vi "oa_Process Order Power Spectrum (N Channels).vi"(0 "even angle signals":cluster{"r0":dbl, "dr":dbl, "Y":dbl[]}[](array[cluster]) {"r0" format="%.2p"; "dr" format="%.2p"; "Y" format="%.2f"}, 5 "channel info":T9[](array[typedef]) {"channel info"."pregain" format="%.2f"; "channel info"."weighting filter" items=["Linear", "A-weighting", "B-weighting", "C-weighting", "ITU-R 468-4", "Dolby", "CCITT", "C-message", "Wb", "Wc", "Wd", "We", "Wf", "Wh", "Wj", "Wk", "Wm", "AES17 20 kHz lowpass", "AES17 40 kHz lowpass", "AES17 20 kHz highpass", "AES17 40 kHz highpass"]; "channel info"."dB reference" format="%^.1e"; "channel info"."engineering units" items=["custom..."=0, "V"=1, "A"=21, "C"=30, "pC"=31, "s"=32, "-"=29, "Pa"=2, "N"=20, "g"=3, "m/s^2"=4, "m/s"=5, "m"=6, "mm/s"=12, "mm"=13, "micron/s"=14, "micron"=15, "in/s^2"=7, "in/s"=8, "in"=9, "mil/s"=10, "mil"=11, "rad/s^2"=16, "rad/s"=17, "rad"=18, "deg/s^2"=26, "deg/s"=27, "deg"=28, "RPM"=22, "cycle/s^2"=23, "Hz"=24, "cycle"=25, "strain"=19]; "channel info"."sensor sensitivity" format="%#_5f"}, 7 "spectrum settings":cluster{"window type":u32, "block size":i32}={"window type"=1, "block size"=400} {"block size" min=2; "window type" items=["None"=0, "Hanning"=1, "Hamming"=2, "Blackman-Harris"=3, "Exact Blackman"=4, "Blackman"=5, "Flat Top"=6, "4 Term B-Harris"=7, "7 Term B-Harris"=8, "Low Sidelobe"=9, "Gaussian"=62]}, 9 "averaging parameters":T11={"averaging mode"=enum."No averaging", "weighting mode"=enum."Exponential", "number of averages"=10, "linear mode"=enum."One shot"} {"number of averages" min=1 step=1}, 11 "error in":errorcluster, 12 "processing control in":T8(ring)) -> (2 "new spectrum available?":bool, 3 "averages completed":dbl, 4 "order power spectrum":T7(array[cluster]) {"order 0" format="%.2p"; "delta order" format="%.2p"; "magnitude" format="%.2f"}, 8 "averaging done":bool, 10 "spectrum info":T1[](array[typedef]) {"x-axis units" items=["Time (s)"=0, "Frequency-CB (Hz)"=1, "Frequency-CPB (Hz)"=1248, "Frequency-Arbitrary (Hz)"=2357, "Quefrency (s)"=2, "Revolutions (rev)"=3, "Order"=4, "Speed (RPM)"=11, "Speed (rad/s)"=21, "Index"=65535]; "weighting filter" items=["Linear", "A-weighting", "B-weighting", "C-weighting", "ITU-R 468-4", "Dolby", "CCITT", "C-message", "Wb", "Wc", "Wd", "We", "Wf", "Wh", "Wj", "Wk", "Wm", "AES17 20 kHz lowpass", "AES17 40 kHz lowpass", "AES17 20 kHz highpass", "AES17 40 kHz highpass"]; "dB reference [EU]" format="%.2f"; "engineering units" items=["custom..."=0, "V"=1, "A"=21, "C"=30, "pC"=31, "s"=32, "-"=29, "Pa"=2, "N"=20, "g"=3, "m/s^2"=4, "m/s"=5, "m"=6, "mm/s"=12, "mm"=13, "micron/s"=14, "micron"=15, "in/s^2"=7, "in/s"=8, "in"=9, "mil/s"=10, "mil"=11, "rad/s^2"=16, "rad/s"=17, "rad"=18, "deg/s^2"=26, "deg/s"=27, "deg"=28, "RPM"=22, "cycle/s^2"=23, "Hz"=24, "cycle"=25, "strain"=19]; "spectral info"."window" items=["None "=0, "Hanning"=1, "Hamming"=2, "Blackman-Harris"=3, "Exact Blackman"=4, "Blackman"=5, "Flat Top"=6, "4 Term B-Harris "=7, "7 Term B-Harris"=8, "Low Sidelobe"=9, "Force - Exponential"=10, "Gaussian"=62]}, 14 "processing control out":T8(ring), 15 "error out":errorcluster)   [LabVIEW 2017, in "SoundVib_Resampling.lvlib"]
uses:
  <vilib>/addons/Sound and Vibration/Order Analysis/Resample Order Tracking/SoundVib_Resampling.lvlib
  <vilib>/addons/_NISVFA/_Shared subVIs/Controls/svc_Resampled Channel Info.ctl
  <vilib>/addons/_NISVFA/_Shared subVIs/Controls/svc_Channel Info.ctl
  <vilib>/addons/_NISVFA/_Shared subVIs/Controls/svc_Engineering Units Text Ring.ctl
  <vilib>/addons/_NISVFA/_Shared subVIs/Controls/svc_Weighting Filter Text Ring.ctl
  <vilib>/addons/_NISVFA/_Shared subVIs/Controls/svc_Spectrum Info.ctl
  <vilib>/addons/_NISVFA/_Shared subVIs/Controls/svc_X-Axis Units.ctl
  <vilib>/addons/_NISVFA/_Shared subVIs/Controls/svc_Spectrum Type.ctl
  <vilib>/addons/_NISVFA/_Shared subVIs/Controls/svc_Complimentary Spectrum Units.ctl
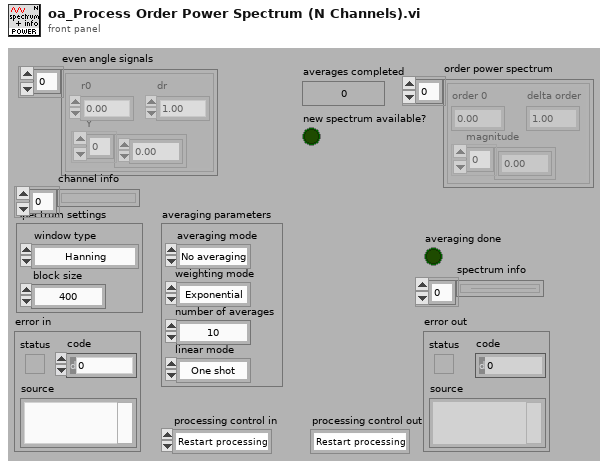
[diagram p1: front panel]
types:
  T1 = typedef "svc_Spectrum Info.ctl" = cluster{"channel name":string, "description":string, "x-axis units":T2, "spectral info":cluster{"spectrum type":T3, "linear/dB":enum16{"linear", "dB"}, "window":u16, "window size":i32, "FFT size":i32}, "engineering units":T4, "custom label":string, "dB reference [EU]":dbl, "peak units":enum16{"rms", "peak", "peak-peak"}, "weighting filter":T5, "spectral density?":bool, "unit label":string, "spectrum skewed?":bool, "complimentary spectrum units":T6}
  T2 = typedef "svc_X-Axis Units.ctl" = u16
  T3 = typedef "svc_Spectrum Type.ctl" = enum16{"FFT Spectrum [complex]", "Amplitude [Magnitude]", "Power [Magnitude^2]", "Cross Spectrum [complex]", "Frequency Response [Complex]"}
  T4 = typedef "svc_Engineering Units Text Ring.ctl" = u16
  T5 = typedef "svc_Weighting Filter Text Ring.ctl" = u16
  T6 = typedef "svc_Complimentary Spectrum Units.ctl" = enum16{"none", "radians", "degrees", "cycles", "imaginary"}
  T7 = cluster{"order 0":dbl, "delta order":dbl, "magnitude":dbl[]}[]
  T8 = enum16{"Restart processing", "Continue processing", "Skip processing"}
  T9 = typedef "svc_Resampled Channel Info.ctl" = cluster{"channel name":string, "description":string, " channel info":T10}
  T10 = typedef "svc_Channel Info.ctl" = cluster{"sensor sensitivity":dbl, "engineering units":T4, "dB reference":dbl, "custom label":string, "weighting filter":T5, "pregain":dbl}
  T11 = cluster{"averaging mode":enum16{"No averaging", "Vector averaging", "RMS averaging", "Peak hold"}, "weighting mode":enum16{"Linear", "Exponential"}, "number of averages":u32, "linear mode":enum16{"One shot", "Auto restart"}}
  T12 = cluster{"complex FFT":cdb[], "power spectrum":dbl[], "averages completed":dbl}[]
  T13 = enum16{"No averaging", "Vector averaging", "RMS averaging", "Peak hold"}
  T14 = cluster{"complex FFT":cdb[], "power spectrum":dbl[], "averages completed":dbl}
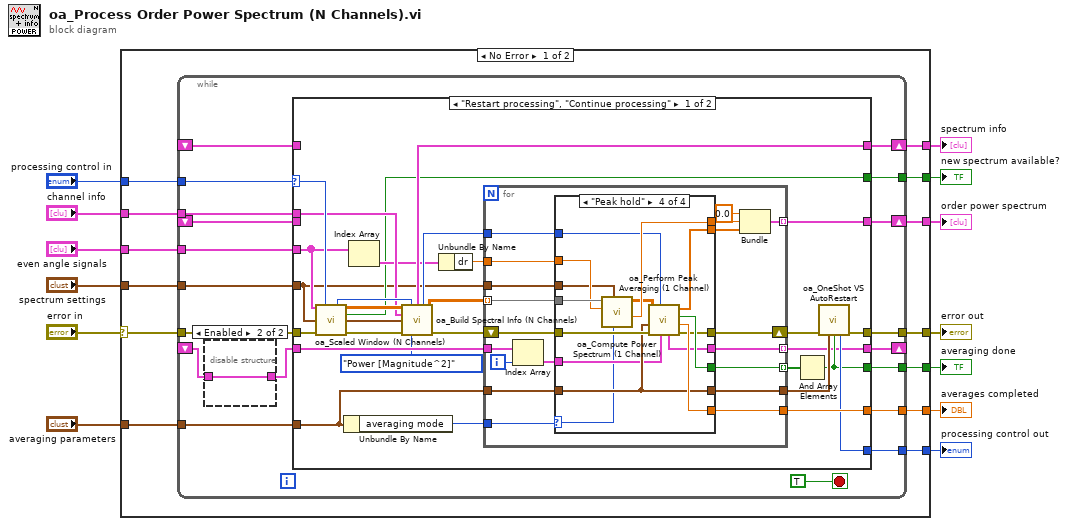
[diagram p0: block diagram]
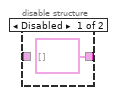
[diagram p2: hidden frame]
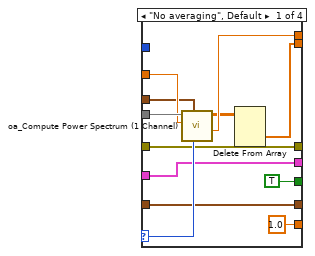
[diagram p3: hidden frame]
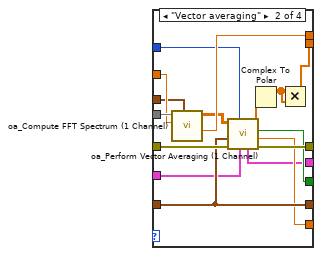
[diagram p4: hidden frame]
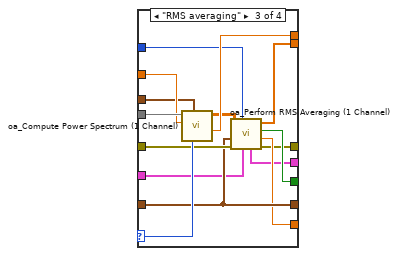
[diagram p5: hidden frame]
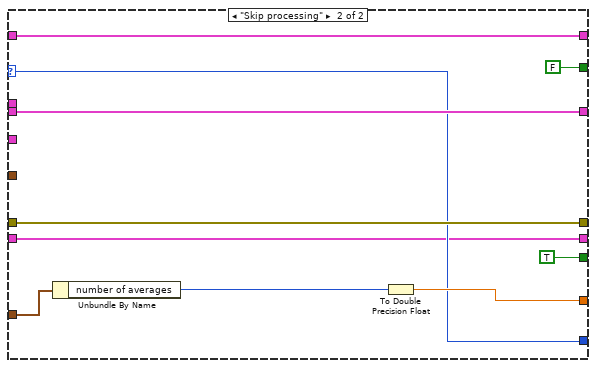
[diagram p6: hidden frame]
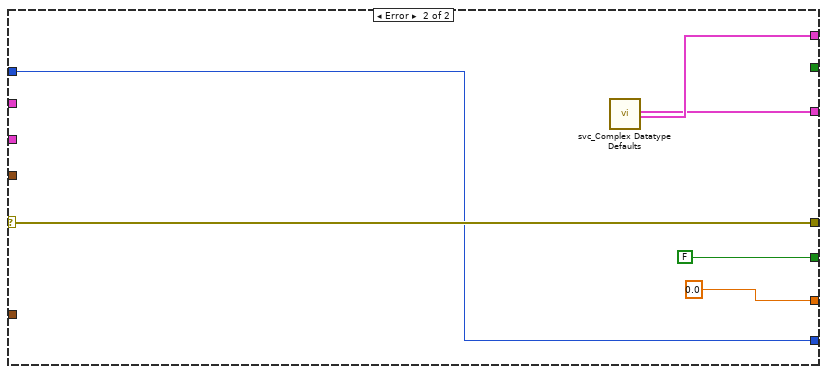
[diagram p7: hidden frame]
diagram:
  n1 = case shown="No Error" "error in" {
    selector: "error in" -> [w25 w169]
    tunnel: [w19 w169] -> w12
    tunnel: "even angle signals" -> [w26 _]
    tunnel: "spectrum settings" -> [w24 _]
    tunnel: "processing control in" -> [w23 w166]
    tunnel: "channel info" -> [w22 _]
    tunnel: "averaging parameters" -> [w21 _]
    tunnel: [w20 w165] -> w2
    tunnel: [w18 0.0 ("averages completed")] -> w6
    tunnel: [w17 FALSE ("averaging done")] -> w5
    tunnel: [w16 w164] -> w3
    tunnel: [w15 w166] -> w4
    tunnel: [w14 _] -> w1
    frame No Error {
      n2 = while {
        tunnel: w26 -> [w44]
        tunnel: w25 -> [w43]
        tunnel: w24 -> [w42]
        tunnel: w23 -> [w41]
        tunnel: w22 -> [w40]
        tunnel: w21 -> [w39]
        shift-right: [w38] -> w20
        shift-left: _ -> [w37]
        tunnel: [w36] -> w19
        tunnel: [w35] -> w18
        tunnel: [w34] -> w17
        shift-right: [w33] -> w16
        shift-left: _ -> [w32]
        tunnel: [w31] -> w15
        shift-right: [w30] -> _
        shift-left: _ -> [w27]
        tunnel: [w29] -> w14
        stop <- TRUE stop-if-true
        n3 = disable-structure shown="Enabled" {
          disable-tunnel: [T12 [] w47] -> w28
          disable-tunnel: w27 -> [_ w47]
          frame Disabled {
          }
          frame Enabled {
          }
        }
        n4 = case shown="\"Restart processing\", \"Continue processing\"" w41 {
          selector: w41 -> [w75 w156]
          tunnel: w44 -> [w52 _]
          tunnel: w43 -> [w76 w162]
          tunnel: w42 -> [w48 _]
          tunnel: w40 -> [w56 _]
          tunnel: w39 -> [w66 w160]
          tunnel: [w68 w163] -> w38
          tunnel: w37 -> [_ w163]
          tunnel: [w62 w162] -> w36
          tunnel: [w65 w158] -> w35
          tunnel: [w57 TRUE ("averaging done")] -> w34
          tunnel: [w64 w157] -> w33
          tunnel: w32 -> [_ w157]
          tunnel: [w59 w156] -> w31
          tunnel: [w55 w155] -> w30
          tunnel: w28 -> [w54 w155]
          tunnel: [w49 FALSE ("new spectrum available?")] -> w29
          frame "Restart processing", "Continue processing" {
            n5 = call <vilib>:"oa_Scaled Window (N Channels).vi"("resampled signals"=w52, "processing control in"=w75, "spectrum settings"=w48, "error in"=w76) -> ("dup processing control"=w72:T8, "Y"=w58:dbl[][][], "new spectrum available?"=w49:bool, "spectrum settings out"=w73:cluster{"window type":u32, "block size":i32}, "error out"=w74:errorcluster)  [unwired: 7 in]
            n6 = Unbundle By Name(w66) -> ("averaging mode"=w71:T13)
            n7 = Index Array(array=w52) -> (element=w51:cluster{"r0":dbl, "dr":dbl, "Y":dbl[]})  [unwired: 1 in]
            n8 = call <vilib>:"oa_Build Spectral Info (N Channels).vi"("spectra in"=w58, "processing control in"=w72, "channel info"=w56, "spectrum settings"=w73, "error in"=w74, "spectrum type"=svc_Spectrum_Type."Power [Magnitude^2]") -> ("spectrum info"=w68:T1[], "dup processing control"=w67:T8, "spectra out"=w70:dbl[][][], "error out"=w69:errorcluster)  [unwired: 6 in]
            n9 = Unbundle By Name(w51) -> ("dr"=w50:dbl)
            n10 = for {
              tunnel: w71 -> [w95]
              tunnel: w70 -> [w94] mode=indexing
              tunnel: w67 -> [w83]
              tunnel: w66 -> [w92]
              tunnel: [w91] -> w65
              tunnel: [w87] -> w64 mode=indexing
              tunnel: [w85] -> w61
              tunnel: [w84] -> w60 mode=indexing
              shift-right: [w86] -> w63
              shift-left: w69 -> [w93]
              tunnel: [w82] -> w55 mode=indexing
              tunnel: w54 -> [w81]
              tunnel: w50 -> [w78]
              tunnel: w48 -> [w77]
              i -> [w80]
              n11 = Index Array(array=w81, index=w80) -> (element=w79:T14)
              n12 = case shown="\"Peak hold\"" w95 {
                selector: w95 -> [w105 _ w136 w140]
                tunnel: w94 -> [w107 w123 w138 w153]
                tunnel: w93 -> [w104 w118 w133 w144]
                tunnel: w83 -> [_ w119 w131 w149]
                tunnel: w78 -> [w106 w122 w137 w152]
                tunnel: [w96 w108 w130 w148] -> w90
                tunnel: [w104 w116 w127 w145] -> w86
                tunnel: w92 -> [w100 w117 w132 w143]
                tunnel: [1.0 ("averages completed") w115 w128 w146] -> w91
                tunnel: [TRUE ("averaging done") w114 w129 w147] -> w84
                tunnel: [w103 w121 w135 w151] -> w88
                tunnel: [w100 w117 w132 w143] -> w85
                tunnel: [w99 w113 w126 w142] -> w82
                tunnel: w79 -> [w99 w112 w125 w141]
                tunnel: w77 -> [w98 w111 w124 w139]
                frame "No averaging", Default {
                  n13 = call <vilib>:"oa_Compute Power Spectrum (1 Channel).vi"("averaging mode"=w105, "spectrum settings"=w98, "dr"=w106, "Y"=w107) -> ("df"=w103:dbl, "power spectrum"=w97:dbl[][])  [unwired: 6 in]
                  n14 = Delete From Array(array=w97) -> (deleted portion=w96:dbl[])  [unwired: 3 in, 1 out]
                }
                frame "Vector averaging" {
                  n15 = call <vilib>:"oa_Compute FFT Spectrum (1 Channel).vi"("spectrum settings"=w111, "dr"=w122, "Y"=w123) -> ("df"=w121:dbl, "one-sided FFT spectrum"=w120:cdb[][])  [unwired: 7 in]
                  n16 = call <vilib>:"oa_Perform Vector Averaging (1 Channel).vi"("averaging state info in"=w112, "processing control in"=w119, "error in (no error)"=w118, "averaging parameters"=w117, "Y"=w120) -> ("error out"=w116:errorcluster, "averages completed"=w115:dbl, "averaging done"=w114:bool, "Y out"=w109:cdb[], "averaging state info out"=w113:T14)  [unwired: 2 in]
                  n17 = Complex To Polar(r * e^(i*theta)=w109) -> (r=w110:dbl[])  [unwired: 1 out]
                  n18 = Multiply(x=w110, y=w110) -> (x*y=w108:dbl[])
                }
                frame "RMS averaging" {
                  n19 = call <vilib>:"oa_Compute Power Spectrum (1 Channel).vi"("averaging mode"=w136, "spectrum settings"=w124, "dr"=w137, "Y"=w138) -> ("df"=w135:dbl, "power spectrum"=w134:dbl[][])  [unwired: 6 in]
                  n20 = call <vilib>:"oa_Perform RMS Averaging (1 Channel).vi"("averaging state info in"=w125, "processing control in"=w131, "error in (no error)"=w133, "averaging parameters"=w132, "Y"=w134) -> ("error out"=w127:errorcluster, "averages completed"=w128:dbl, "averaging done"=w129:bool, "Y out"=w130:dbl[], "averaging state info out"=w126:T14)  [unwired: 2 in]
                }
                frame "Peak hold" {
                  n21 = call <vilib>:"oa_Compute Power Spectrum (1 Channel).vi"("averaging mode"=w140, "spectrum settings"=w139, "dr"=w152, "Y"=w153) -> ("df"=w151:dbl, "power spectrum"=w150:dbl[][])  [unwired: 6 in]
                  n22 = call <vilib>:"oa_Perform Peak Averaging (1 Channel).vi"("averaging state info out"=w141, "processing control in"=w149, "error in (no error)"=w144, "averaging parameters"=w143, "Y"=w150) -> ("error out"=w145:errorcluster, "averages completed"=w146:dbl, "averaging done"=w147:bool, "Y out"=w148:dbl[], "averaging state info out"=w142:T14)  [unwired: 2 in]
                }
              }
              n23 = Bundle(0.0, "df"=w88, "Y out"=w90) -> (w87:cluster{dbl, "df":dbl, "Y out":dbl[]})  [unwired: 1 in]
            }
            n24 = And Array Elements(Boolean array=w60) -> (logical AND=w57:bool)
            n25 = call <vilib>:"oa_OneShot VS AutoRestart.vi"("error in (no error)"=w63, "averaging parameters"=w61, "averaging done"=w57) -> ("processing control out"=w59:T8, "error out"=w62:errorcluster)  [unwired: 11 in]
          }
          frame "Skip processing" {
            n26 = Unbundle By Name(w160) -> ("number of averages"=w159:u32)
            n27 = To Double Precision Float(number=w159) -> (double precision float=w158:dbl)
          }
        }
      }
    }
    frame Error {
      n28 = call <vilib>:"svc_Complex Datatype Defaults.vi"() -> ("empty array of spectra"=w164:cluster{"f0":dbl, "df":dbl, "magnitude":dbl[]}[], "empty array of spectrum info"=w165:T1[])  [unwired: 11 in, 7 out]
    }
  }
  "error out" <- w12
  "averaging done" <- w5
  "averages completed" <- w6
  "processing control out" <- w4
  "order power spectrum" <- w3
  "spectrum info" <- w2
  "new spectrum available?" <- w1
